vi "Path Track Loop.vi"(8 "error in":errorcluster) -> ()   [LabVIEW 2016, in "Path Track.lvlib"]
uses:
  Path Track.lvlib
panel:
  out "Chart 2":dbl(graph)
  in  "Get ms ago":u32=60
  in  "Enable Test?":bool
  out "Chart":cluster{"Angle":dbl, "Angle":dbl}(graph)
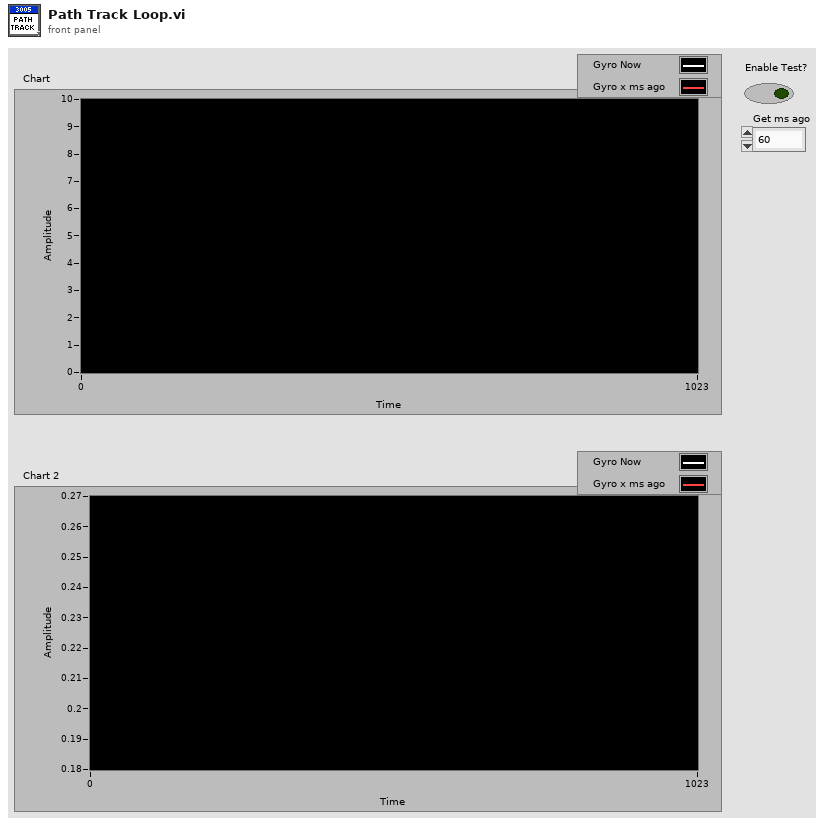
[diagram p1: front panel]
types:
  T1 = typedef "WPI_GyroDevRef.ctl" = cluster{"DevStatus":errorcluster, "Analog Channel":T2, "Offset":dbl, "Gain (VoltsPerDegree/Second)":dbl, "Gyro Type":enum16{"Analog", "XRS450"}, "Handle":i32, "SPI Bus":T3, "Device Found":bool, "Sample Rate":dbl, "Calibrate On Open":bool}
  T2 = typedef "FPGA_AIChannel.ctl" = enum8{"AI 0", "AI 1", "AI 2", "AI 3", "AI MXP 0", "AI MXP 1", "AI MXP 2", "AI MXP 3", "Invalid"}
  T3 = typedef "spi_bus.ctl" = enum16{"SPI On-Board, CS0", "SPI On-Board, CS1", "SPI On-Board, CS2", "SPI On-Board, CS3", "SPI MXP", "Invalid"}
  T4 = typedef "WPI_AnalogChannelDevRef.ctl" = cluster{"DevStatus":errorcluster, "Analog Channel":T2}
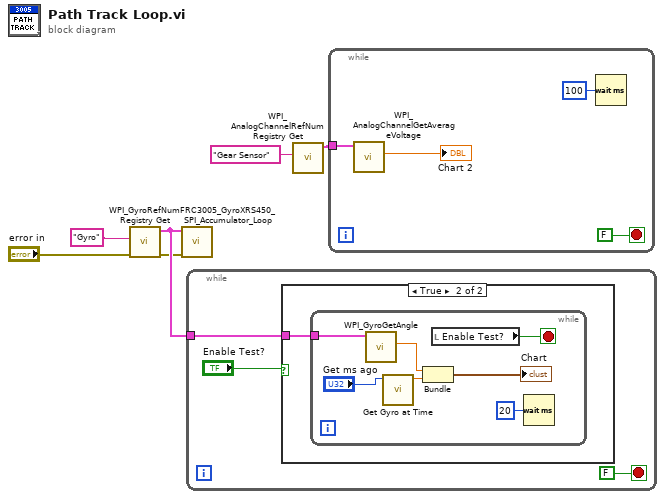
[diagram p0: block diagram]
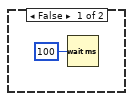
[diagram p2: hidden frame]
diagram:
  n1 = call <vilib>:"WPI_GyroRefNum Registry Get.vi"("error in (no error)"="error in", "refnum name"="Gyro") -> ("error out"=w2:errorcluster, "GyroDevRef"=w5:T1)  [unwired: 8 in]
  n2 = call "FRC3005_GyroXRS450_SPI_Accumulator_Loop.vi"("error in"=w2, "GyroDeviceRef"=w5) -> ()  [unwired: 9 in, 1 out]
  n3 = while {
    tunnel: w5 -> [w9]
    stop <- FALSE stop-if-true
    n4 = case shown="True" "Enable Test?" {
      tunnel: w9 -> [_ w11]
      frame False {
        n5 = Wait (ms)(milliseconds to wait=u32 100) -> ()  [unwired: 1 out]
      }
      frame True {
        n6 = while {
          tunnel: w11 -> [w15]
          stop <- w12 stop-if-true
          n7 = call <vilib>:"WPI_GyroGetAngle.vi"("GyroDevRef"=w15) -> ("Angle"=w14:dbl)  [unwired: 6 in, 4 out]
          n8 = call "Get Gyro at Time.vi"("Get ms ago"="Get ms ago") -> ("Angle"=w16:dbl)  [unwired: 9 in, 1 out]
          n9 = Bundle("Angle"=w14, "Angle"=w16) -> (→"Chart":cluster{"Angle":dbl, "Angle":dbl})  [unwired: 1 in]
          n10 = local read "Enable Test?"() -> (w12:bool)
          n11 = Wait (ms)(milliseconds to wait=u32 20) -> ()  [unwired: 1 out]
        }
      }
    }
  }
  n12 = call <vilib>:"WPI_AnalogChannelRefNum Registry Get.vi"("refnum name"="Gear Sensor") -> ("AIDeviceRef"=w3:T4)  [unwired: 9 in, 1 out]
  n13 = while {
    tunnel: w3 -> [w21]
    stop <- FALSE stop-if-true
    n14 = call <vilib>:"WPI_AnalogChannelGetAverageVoltage.vi"("AIDeviceRef"=w21) -> ("Voltage"=→"Chart 2":dbl)  [unwired: 8 in, 2 out]
    n15 = Wait (ms)(milliseconds to wait=u32 100) -> ()  [unwired: 1 out]
  }
